vi "Stop Core.vi"(10 "final error code":i32, 11 "CS++DCPwr in":refnum<class "CS++DCPwr.lvclass">) -> (3 "CS++DCPwr out":refnum<class "CS++DCPwr.lvclass">)   [LabVIEW 2013, in "CS++DCPwr.lvlib" / "CS++DCPwr.lvclass"]
doc: "(<B>Filename</B>: Actor Framework.lvlib:Actor.lvclass:Stop Core.vi)\n\nDefines what the actor does before it stops. Use the <B>final error code</B> input to determine whether the actor shut down in response to an error.\n\nBy default, this method does nothing. A descendant class may override it to define behavior, such as shutting down any processes the actor initiated in its override of the Actor Core method."
uses:
  CS++DCPwr.lvclass
  <vilib>/ActorFramework/Time-Delayed Send Message/Time-Delay Override Options.ctl
  CSPP_Core/Actors/CS++DeviceActor/CS++DeviceActor.lvclass
  CS++DCPwr.lvclass/CS++DCPwr.ctl
  CSPP_Core/Classes/CS++ProcessVariables/PVConnection/PVConnection.lvclass
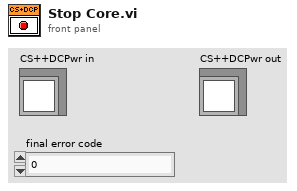
[diagram p1: front panel]
types:
  T1 = typedef "Time-Delay Override Options.ctl" = enum16{"Send next copy now", "Skip next scheduled copy", "Send next copy now and stop all further copies", "Stop all further copies"}
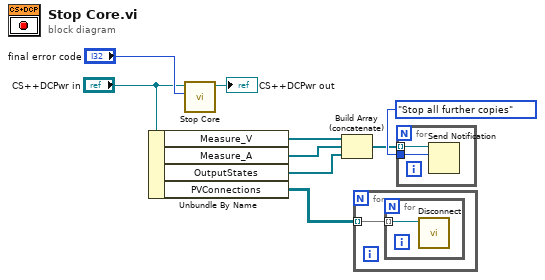
[diagram p0: block diagram]
diagram:
  n1 = Unbundle By Name("CS++DCPwr in") -> ("Measure_V"=w6:refnum<notifier>[], "Measure_A"=w3:refnum<notifier>[], "OutputStates"=w2:refnum<notifier>[], "PVConnections"=w1:refnum<class "PVConnection.lvclass">[][])
  n2 = call-parent "Stop Core.vi"("final error code"="final error code", "CS++DeviceActor in"="CS++DCPwr in") -> ("CS++DeviceActor out"=→"CS++DCPwr out":refnum<class "CS++DCPwr.lvclass">)  [unwired: 9 in]
  n3 = Build Array (concatenate)(w6, w3, w2) -> (w4:refnum<notifier>[])
  n4 = for {
    tunnel: w1 -> [w10] mode=indexing
    n5 = for {
      tunnel: w10 -> [w11] mode=indexing
      n6 = call-dynamic "Disconnect.vi"("PVConnection in"=w11) -> ()  [unwired: 9 in, 2 out]
    }
  }
  n7 = for {
    tunnel: w4 -> [w13] mode=indexing
    tunnel: Time-Delay_Override_Options."Stop all further copies" ("notification") -> [w12]
    n8 = Send Notification(notification=w12, notifier=w13) -> ()  [unwired: 1 in, 2 out]
  }
